vi "LoggingState.vi"() -> ()   [LabVIEW 2020]
uses:
  <vilib>/Skyline/Tag/Shared/typedefs/DataType.ctl
  <vilib>/Skyline/Configuration/Configuration HTTP_class/NI Skyline Configuration HTTP.lvclass/NI Skyline Configuration HTTP.ctl
  <vilib>/Skyline/Configuration/Configuration HTTP_class/Open Configuration HTTP.vi
  <vilib>/Skyline/Configuration/HTTP/Open Configuration (Desktop).vi
  <vilib>/Skyline/Tag/Wrapper/Wrapper HTTP_class/Open Tag HTTP.vi
  <vilib>/Skyline/Tag/Wrapper/Wrapper_class/Write Tag (String).vi
  <vilib>/Skyline/Tag/Wrapper/Wrapper_class/Delete Tag (Single).vi
  <vilib>/Skyline/Configuration/Configuration HTTP_class/NI Skyline Configuration HTTP.lvclass
  <vilib>/Skyline/Configuration/Configuration_class/NI Skyline Configuration.lvclass
  <vilib>/Skyline/Tag/Wrapper/Wrapper_class/NI Skyline Tag.lvclass
  <vilib>/Skyline/Tag/Wrapper/Wrapper HTTP_class/NI Skyline Tag HTTP.lvclass
  <vilib>/Skyline/Tag/Shared/NI Skyline Tag.lvlib
  <vilib>/Skyline/Utilities/NI Skyline Utilities.lvlib
panel:
  in  "stop":bool
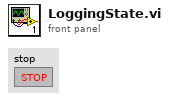
[diagram p1: front panel]
types:
  T1 = typedef "NI Skyline Tag.lvlib/DataType.ctl" = enum32{"Double", "I32", "String", "Boolean", "U64", "Timestamp"}
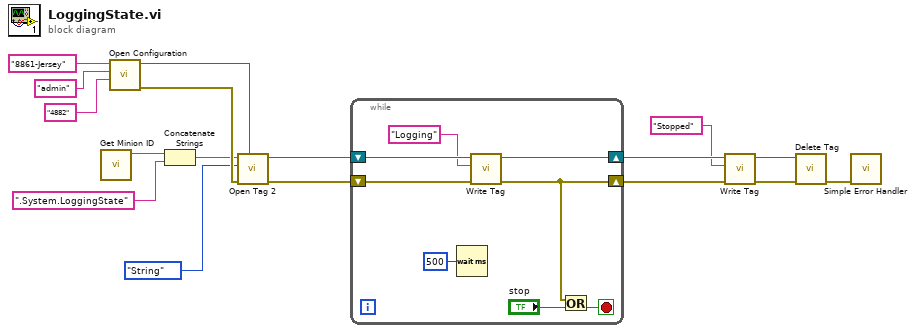
[diagram p0: block diagram]
diagram:
  n1 = call <vilib>:"Get Minion ID.vi"() -> ("minion id"=w10:string)  [unwired: 11 in]
  n2 = call-poly <vilib>:"Open Configuration.vi"("password"="4882" ("server url"), "username"="admin" ("server url"), "server url"="8861-Jersey") -> ("error out"=w16:errorcluster, "configuration"=w17:refnum<class "NI Skyline Configuration HTTP.lvclass">)  [unwired: 7 in]
  n3 = Concatenate Strings(w10, ".System.LoggingState" ("server url")) -> (w9:string)
  n4 = call-poly <vilib>:"Open Tag 2.vi"("configuration"=w17, "error in (no error)"=w16, "Data Type"=DataType."String", "path"=w9) -> ("error out"=w7:errorcluster, "tag"=w8:refnum<class "NI Skyline Tag.lvclass">)  [unwired: 6 in]
  n5 = while {
    shift-right: [w21] -> w5
    shift-left: w8 -> [w25]
    shift-right: [w18] -> w6
    shift-left: w7 -> [w24]
    stop <- w19 stop-if-true
    n6 = Wait (ms)(milliseconds to wait=u32 500) -> ()  [unwired: 1 out]
    n7 = call-poly <vilib>:"Write Tag.vi"("error in (no error)"=w24, "value"="Logging", "tag in"=w25) -> ("error out"=w18:errorcluster, "tag out"=w21:refnum<class "NI Skyline Tag.lvclass">)  [unwired: 7 in]
    n8 = Or(x=w18, y="stop") -> (x .or. y?=w19:bool)
  }
  n9 = call-poly <vilib>:"Write Tag.vi"("error in (no error)"=w6, "value"="Stopped", "tag in"=w5) -> ("error out"=w4:errorcluster, "tag out"=w3:refnum<class "NI Skyline Tag.lvclass">)  [unwired: 7 in]
  n10 = call-poly <vilib>:"Delete Tag.vi"("error in (no error)"=w4, "tag"=w3) -> ("error out"=w2:errorcluster)  [unwired: 9 in]
  n11 = call <vilib>:"Simple Error Handler.vi"("error in (no error)"=w2) -> ()  [unwired: 4 in, 5 out]
